vi "mlink_func_read.vi"(8 "error in (no error)":errorcluster, 10 "function key":enum8{"None", "F1", "F2"}(ring)=enum."F1", 11 "connection ID":i32=-1) -> (0 "error out":errorcluster, 2 "state":bool, 3 "link_fd out":i32)   [LabVIEW 2009, in "MicroDAQ.lvlib" / "mlink.lvlib"]
doc: "This function reads F1/F2 function key state. The function read key and stores its state in \nvariable pointed by state."
uses:
  <instrlib>/MicroDAQ/Mlink library wraper/mlink.lvlib
  <instrlib>/MicroDAQ/MLink32.dll
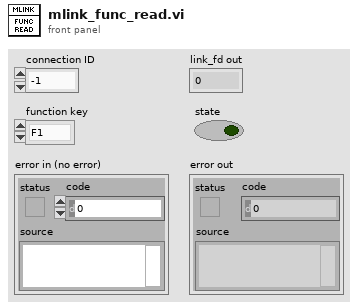
[diagram p1: front panel]
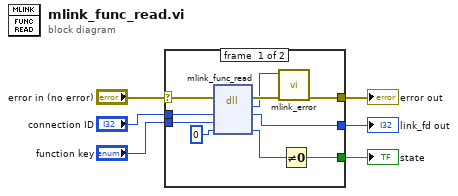
[diagram p0: block diagram]
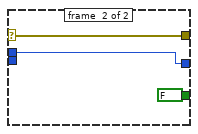
[diagram p2: hidden frame]
diagram:
  n1 = case shown="No Error" "error in (no error)" {
    selector: "error in (no error)" -> [w13 w19]
    tunnel: "connection ID" -> [w16 w18]
    tunnel: [w15 w18] -> w5
    tunnel: [w11 FALSE] -> w3
    tunnel: "function key" -> [w10 _]
    tunnel: [w9 w19] -> w1
    frame #0 {
      n2 = dll-call lib="C:/Program Files (x86)/National Instruments/LabVIEW 2009/instr.lib/MicroDAQ/MLink32.dll" fn="mlink_func_read"(error in=w13, "link_fd"=w16, "key"=w10, "state"=u8 0) -> (error out=w8:errorcluster, "return type"=w7:i32, "link_fd"=w15:i32, "state"=w12:u8)  [unwired: 3 in, 1 out]
      n3 = call <instrlib>:"mlink_error.vi"("error in (no error)"=w8, "error code"=w7) -> ("error out"=w9:errorcluster)  [unwired: 9 in]
      n4 = Not Equal To 0?(x=w12) -> (x != 0?=w11:bool)
    }
    frame #1 {
    }
  }
  "link_fd out" <- w5
  "error out" <- w1
  "state" <- w3
